vi "User Manual Example 2.vi"() -> ()   [LabVIEW 2013]
uses:
  <instrlib>/SRS SR400/Public/Typedefs/Counter.ctl
  <instrlib>/SRS SR400/Public/Typedefs/Counter Input.ctl
  <instrlib>/SRS SR400/Public/Typedefs/Gate Mode.ctl
  <instrlib>/SRS SR400/Public/Typedefs/Discriminator Slope.ctl
  <instrlib>/SRS SR400/Examples/Typedefs/Example 2 Program State.ctl
  <instrlib>/SRS SR400/Public/Typedefs/Menu Display Line.ctl
  <instrlib>/SRS SR400/Public/Typedefs/Status Bit.ctl
  <instrlib>/SRS SR400/SRS SR400.lvlib
panel:
  in  "Discriminator Slope":T1
  in  "Discriminator Level":dbl=0.15
  out "Counts":i16[](array[numeric])
  in  "Gate Width":dbl=0.5
  in  "Gate Delay":dbl=0.5
  in  "Gate Mode":T2=enum."Fixed"
  in  "Dwell Time":dbl=6.0
  in  "Number of Periods":u16=10 max=2000 step=1
  in  "Counter Preset":u64=1
  in  "Counter Input":T3=enum."TRIG"
  in  "Counter":T4=enum."T"
  in  "SRS SR400":refnum<visa-resource-name>
  # "LEVEL Settings"
  # "A GATE Settings"
  # "MODE Settings"
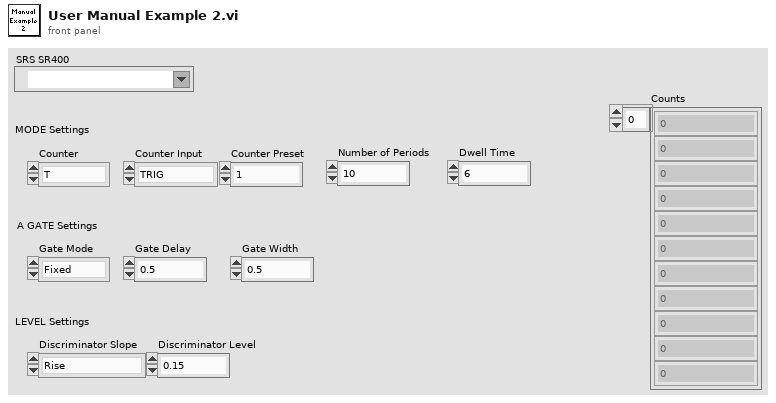
[diagram p1: front panel]
types:
  T1 = typedef "SRS SR400.lvlib/Discriminator Slope.ctl" = enum16{"Rise", "Fall"}
  T2 = typedef "SRS SR400.lvlib/Gate Mode.ctl" = enum16{"CW", "Fixed", "Scan"}
  T3 = typedef "SRS SR400.lvlib/Counter Input.ctl" = enum16{"10 MHz", "INPUT 1", "INPUT 2", "TRIG"}
  T4 = typedef "SRS SR400.lvlib/Counter.ctl" = enum16{"A", "B", "T"}
  T5 = typedef "Example 2 Program State.ctl" = enum16{"Initialize", "Set Scan Parameters", "Reset Count", "Start Count", "Check for Data Ready", "Read Count", "Check for Scan Finished", "Close Hardware"}
  T6 = typedef "SRS SR400.lvlib/Menu Display Line.ctl" = enum16{"1,1     COUNT", "1,2     A", "1,3     B", "1,4     T", "1,5     N PERIODS", "1,6     AT N", "1,7     D/A OUT", "1,8     D/A RANGE", "1,9     DISPLAY", "2,1     A GATE", "2,2     A DELAY", "2,3     A WIDTH", "3,1     B GATE", "3,2     B DELAY", "3,3     B WIDTH", "4,1     TRIG SLOPE", "4,2     TRIG LVL", "4,3     A DISC SLOPE", "4,4     A DISC MODE", "4,5     A DISC LVL", "4,6     B DISC SLOPE", "4,7     B DISC MODE", "4,8     B DISC LVL", "4,9     T DISC SLOPE", "4,10   T DISC MODE", "4,11   T DISC LVL", "4,12   PORT1 MODE", "4,13   PORT1 LVL", "4,14   PORT2 MODE", "4,15   PORT2 LVL", "5,1     GPIB ADDR", "5,2     RS-232 BAUD", "5,3     RS-232 BITS", "5,4     RS-232 PARITY", "5,5     RS-232 WAIT", "5,6     RS-232 ECHO", "5,7     DATA", "6,1     LCD CONTRAST", "6,2     STORE", "6,3     RECALL"}
  T7 = typedef "SRS SR400.lvlib/Status Bit.ctl" = enum16{"Parameter Changed", "Data Ready", "Scan Finished", "Counter Overrun", "Rate Error", "Recall Error", "SRQ", "Command Error"}
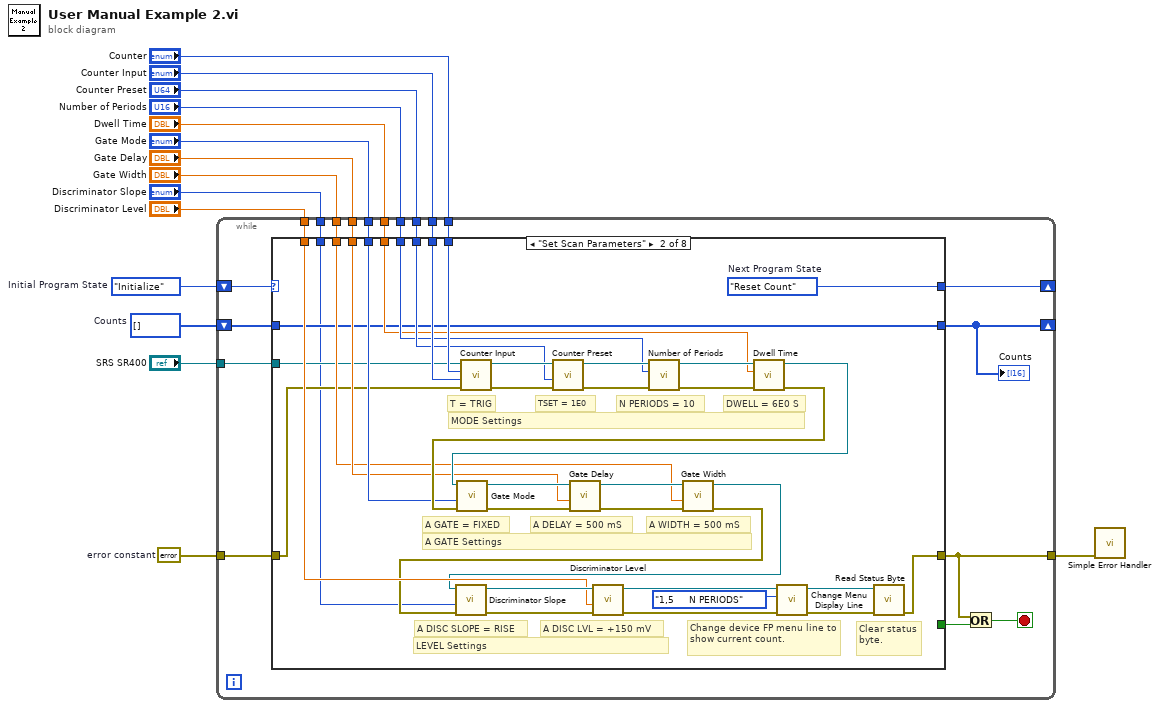
[diagram p0: block diagram]
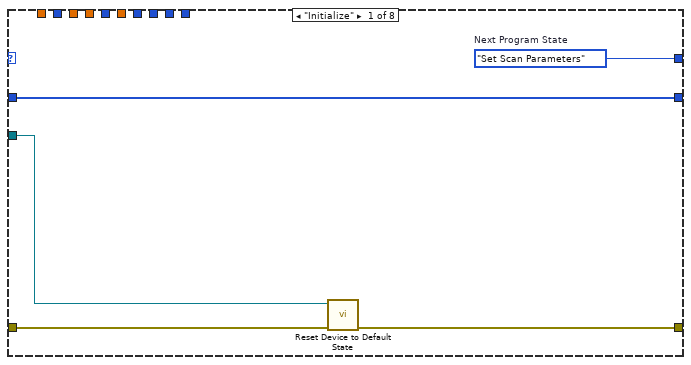
[diagram p2: hidden frame]
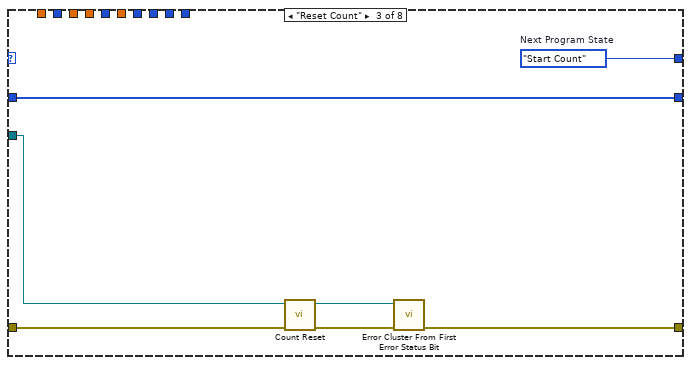
[diagram p3: hidden frame]
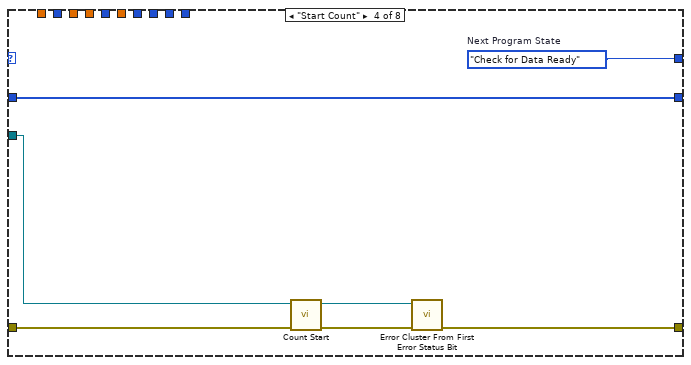
[diagram p4: hidden frame]
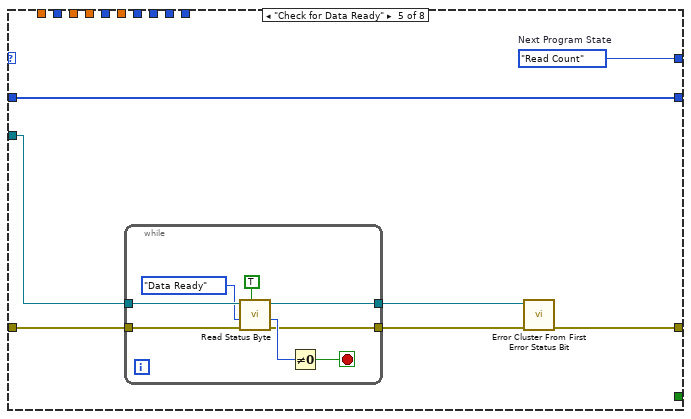
[diagram p5: hidden frame]
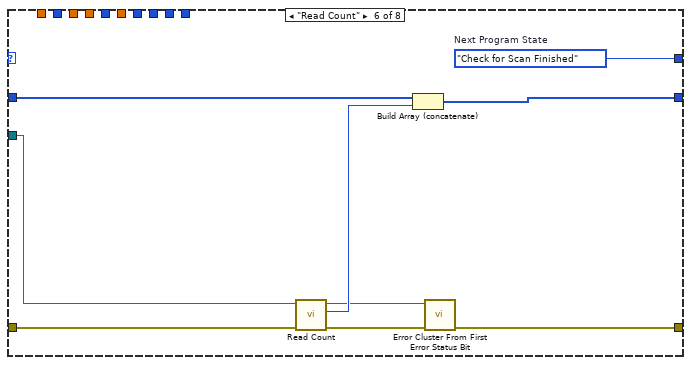
[diagram p6: hidden frame]
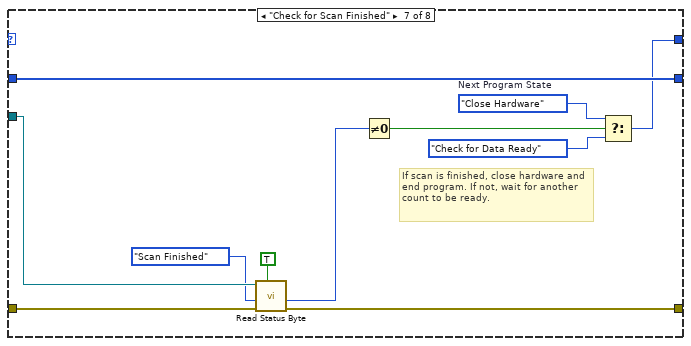
[diagram p7: hidden frame]
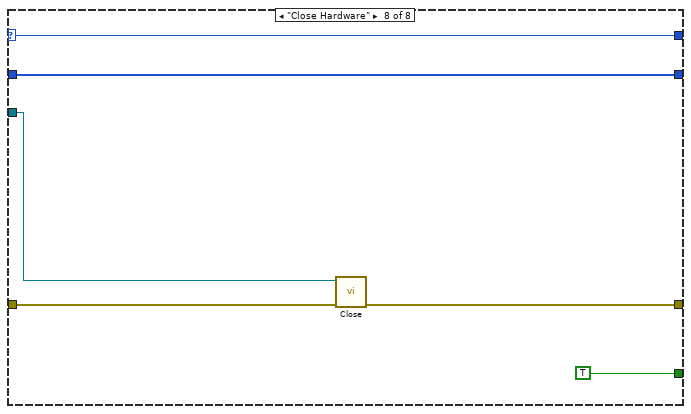
[diagram p8: hidden frame]
diagram:
  w12 = i16[] []  # Counts
  w14 = Example_2_Program_State."Initialize"  # Initial Program State
  w15 = errorcluster {"status"=FALSE, "code"=0, "source"=""}  # error constant
  n1 = while {
    tunnel: w15 -> [w34]
    tunnel: "SRS SR400" -> [w32]
    shift-right: [w19] -> _
    shift-left: w14 -> [w33]
    shift-right: [w18] -> _
    shift-left: w12 -> [w31]
    tunnel: "Counter" -> [w28]
    tunnel: "Counter Input" -> [w27]
    tunnel: "Counter Preset" -> [w26]
    tunnel: "Number of Periods" -> [w25]
    tunnel: "Dwell Time" -> [w24]
    tunnel: "Gate Mode" -> [w23]
    tunnel: "Gate Delay" -> [w22]
    tunnel: "Gate Width" -> [w21]
    tunnel: "Discriminator Level" -> [w20]
    tunnel: [w17] -> w2
    tunnel: "Discriminator Slope" -> [w16]
    stop <- w30 stop-if-true
    n2 = case shown="\"Set Scan Parameters\"" w33 {
      selector: w33 -> [_ _ _ _ _ _ _ w125]
      tunnel: w34 -> [w39 w50 w79 w87 w94 w112 w123 w128]
      tunnel: w32 -> [w38 w51 w80 w86 w93 w111 w121 w127]
      tunnel: w31 -> [w36 w44 w82 w89 w96 w110 w124 w129]
      tunnel: [w35 w42 w76 w83 w92 w106 w122 w126] -> w17
      tunnel: [_ _ _ _ _ _ _ TRUE] -> w29
      tunnel: w28 -> [_ w60 _ _ _ _ _ _]
      tunnel: w27 -> [_ w59 _ _ _ _ _ _]
      tunnel: w26 -> [_ w58 _ _ _ _ _ _]
      tunnel: w25 -> [_ w57 _ _ _ _ _ _]
      tunnel: w24 -> [_ w56 _ _ _ _ _ _]
      tunnel: w23 -> [_ w55 _ _ _ _ _ _]
      tunnel: w22 -> [_ w54 _ _ _ _ _ _]
      tunnel: w21 -> [_ w53 _ _ _ _ _ _]
      tunnel: w20 -> [_ w52 _ _ _ _ _ _]
      tunnel: [w37 w45 w81 w88 w95 w113 w116 w125] -> w19
      tunnel: [w36 w44 w82 w89 w96 w108 w124 w129] -> w18
      tunnel: w16 -> [_ w40 _ _ _ _ _ _]
      frame "Initialize" {
        w37 = Example_2_Program_State."Set Scan Parameters"  # Next Program State
        n3 = call <instrlib>:"Reset Device to Default State.vi"("error in (no error)"=w39, "VISA resource name"=w38) -> ("error out"=w35:errorcluster)  [unwired: 8 in, 1 out]
      }
      frame "Set Scan Parameters" {
        w45 = Example_2_Program_State."Reset Count"  # Next Program State
        # "Clear status byte."
        # "Change device FP menu line to show current count."
        # "DWELL = 6E0 S"
        # "N PERIODS = 10"
        # "LEVEL Settings"
        # "A DISC LVL = +150 mV"
        # "A GATE Settings"
        # "MODE Settings"
        # "A DISC SLOPE = RISE"
        # "A WIDTH = 500 mS"
        # "A DELAY = 500 mS"
        # "A GATE = FIXED"
        # "TSET = 1E0"
        # "T = TRIG"
        n4 = call <instrlib>:"Counter Input.vi"("error in (no error)"=w50, "Counter Input (INPUT 1)"=w59, "Counter (A)"=w60, "VISA resource name"=w51) -> ("error out"=w68:errorcluster, "VISA resource name out"=w62:refnum<visa-resource-name>)  [unwired: 5 in, 1 out]
        n5 = call <instrlib>:"Counter Preset.vi"("error in (no error)"=w68, "Counter Preset (1)"=w58, "VISA resource name"=w62) -> ("error out"=w69:errorcluster, "VISA resource name out"=w63:refnum<visa-resource-name>)  [unwired: 6 in, 1 out]
        n6 = call <instrlib>:"Number of Periods.vi"("error in (no error)"=w69, "Number of Periods (1)"=w57, "VISA resource name"=w63) -> ("error out"=w70:errorcluster, "VISA resource name out"=w64:refnum<visa-resource-name>)  [unwired: 6 in, 1 out]
        n7 = call <instrlib>:"Dwell Time.vi"("error in (no error)"=w70, "Dwell Time (1E0 s)"=w56, "VISA resource name"=w64) -> ("error out"=w75:errorcluster, "VISA resource name out"=w74:refnum<visa-resource-name>)  [unwired: 6 in, 1 out]
        n8 = call <instrlib>:"Gate Mode.vi"("error in (no error)"=w75, "Gate Mode (CW)"=w55, "VISA resource name"=w74) -> ("error out"=w71:errorcluster, "VISA resource name out"=w65:refnum<visa-resource-name>)  [unwired: 6 in, 1 out]
        n9 = call <instrlib>:"Gate Delay.vi"("error in (no error)"=w71, "Gate Delay (0.000E-6 s)"=w54, "VISA resource name"=w65) -> ("error out"=w72:errorcluster, "VISA resource name out"=w66:refnum<visa-resource-name>)  [unwired: 6 in, 1 out]
        n10 = call <instrlib>:"Gate Width.vi"("error in (no error)"=w72, "Gate Width (0.005E-6 s)"=w53, "VISA resource name"=w66) -> ("error out"=w47:errorcluster, "VISA resource name out"=w46:refnum<visa-resource-name>)  [unwired: 6 in, 1 out]
        n11 = call <instrlib>:"Discriminator Slope.vi"("error in (no error)"=w47, "Discriminator Slope (Fall)"=w40, "VISA resource name"=w46) -> ("error out"=w73:errorcluster, "VISA resource name out"=w67:refnum<visa-resource-name>)  [unwired: 6 in, 1 out]
        n12 = call <instrlib>:"Discriminator Level.vi"("error in (no error)"=w73, "Discriminator Level (-0.0100 V)"=w52, "VISA resource name"=w67) -> ("error out"=w49:errorcluster, "VISA resource name out"=w48:refnum<visa-resource-name>)  [unwired: 6 in, 1 out]
        n13 = call <instrlib>:"Change Menu Display Line.vi"("error in (no error)"=w49, "Menu Display Line [Menu,Line] (COUNT)"=Menu_Display_Line."1,5     N PERIODS", "VISA resource name"=w48) -> ("error out"=w43:errorcluster, "VISA resource name out"=w41:refnum<visa-resource-name>)  [unwired: 7 in]
        n14 = call <instrlib>:"Read Status Byte.vi"("error in (no error)"=w43, "VISA resource name"=w41) -> ("error out"=w42:errorcluster)  [unwired: 6 in, 3 out]
      }
      frame "Reset Count" {
        w81 = Example_2_Program_State."Start Count"  # Next Program State
        n15 = call <instrlib>:"Count Reset.vi"("error in (no error)"=w79, "VISA resource name"=w80) -> ("error out"=w78:errorcluster, "VISA resource name out"=w77:refnum<visa-resource-name>)  [unwired: 8 in]
        n16 = call <instrlib>:"Error Cluster From First Error Status Bit.vi"("error in (no error)"=w78, "VISA resource name"=w77) -> ("error out"=w76:errorcluster)  [unwired: 8 in, 1 out]
      }
      frame "Start Count" {
        w88 = Example_2_Program_State."Check for Data Ready"  # Next Program State
        n17 = call <instrlib>:"Count Start.vi"("error in (no error)"=w87, "VISA resource name"=w86) -> ("error out"=w85:errorcluster, "VISA resource name out"=w84:refnum<visa-resource-name>)  [unwired: 8 in]
        n18 = call <instrlib>:"Error Cluster From First Error Status Bit.vi"("error in (no error)"=w85, "VISA resource name"=w84) -> ("error out"=w83:errorcluster)  [unwired: 8 in, 1 out]
      }
      frame "Check for Data Ready" {
        w95 = Example_2_Program_State."Read Count"  # Next Program State
        n19 = while {
          tunnel: w93 -> [w103]
          tunnel: w94 -> [w104]
          tunnel: [w97] -> w90
          tunnel: [w98] -> w91
          stop <- w99 stop-if-true
          n20 = call <instrlib>:"Read Status Byte.vi"("Read Status Bit? (F)"=TRUE, "error in (no error)"=w104, "Status Bit (Scan Finished)"=Status_Bit."Data Ready", "VISA resource name"=w103) -> ("error out"=w97:errorcluster, "Status Bit"=w100:u8, "VISA resource name out"=w98:refnum<visa-resource-name>)  [unwired: 4 in, 1 out]
          n21 = Not Equal To 0?(x=w100) -> (x != 0?=w99:bool)
        }
        n22 = call <instrlib>:"Error Cluster From First Error Status Bit.vi"("error in (no error)"=w90, "VISA resource name"=w91) -> ("error out"=w92:errorcluster)  [unwired: 8 in, 1 out]
      }
      frame "Read Count" {
        w113 = Example_2_Program_State."Check for Scan Finished"  # Next Program State
        n23 = call <instrlib>:"Read Count.vi"("error in (no error)"=w112, "VISA resource name"=w111) -> ("error out"=w107:errorcluster, "Count"=w109:i16, "VISA resource name out"=w105:refnum<visa-resource-name>)  [unwired: 7 in]
        n24 = Build Array (concatenate)(w110, w109) -> (w108:i16[])
        n25 = call <instrlib>:"Error Cluster From First Error Status Bit.vi"("error in (no error)"=w107, "VISA resource name"=w105) -> ("error out"=w106:errorcluster)  [unwired: 8 in, 1 out]
      }
      frame "Check for Scan Finished" {
        w114 = Example_2_Program_State."Close Hardware"  # Next Program State
        # "If scan is finished, close hardware and end program. If not, wait for another count to be ready."
        n26 = call <instrlib>:"Read Status Byte.vi"("Read Status Bit? (F)"=TRUE, "error in (no error)"=w123, "Status Bit (Scan Finished)"=Status_Bit."Scan Finished", "VISA resource name"=w121) -> ("error out"=w122:errorcluster, "Status Bit"=w118:u8)  [unwired: 4 in, 2 out]
        n27 = Not Equal To 0?(x=w118) -> (x != 0?=w117:bool)
        n28 = Select(t=w114, s=w117, f=Example_2_Program_State."Check for Data Ready" ("Program State")) -> (s? t:f=w116:T5)
      }
      frame "Close Hardware" {
        n29 = call <instrlib>:"Close.vi"("error in (no error)"=w128, "VISA resource name"=w127) -> ("error out"=w126:errorcluster)  [unwired: 9 in]
      }
    }
    "Counts" <- w18
    n30 = Or(x=w17, y=w29) -> (x .or. y?=w30:bool)
  }
  n31 = call <vilib>:"Simple Error Handler.vi"("error in (no error)"=w2) -> ()  [unwired: 4 in, 5 out]
